vi "Send Notify Monitor.vi"(7 "Priority":T1 caption="Message Priority (Normal)", 8 "error in (no error)":errorcluster, 11 "Message Enqueuer in":refnum<class "Message Enqueuer.lvclass">) -> (0 "error out":errorcluster, 3 "Message Enqueuer out":refnum<class "Message Enqueuer.lvclass">)   [LabVIEW 2023, in "Monitored Actor.lvlib" / "Notify Monitor Msg.lvclass"]
doc: "Sends the <b>Monitored Actor.lvlib:Notify Monitor Msg.lvclass</b> message.\n\nThis message will call <b>Notify Monitor.vi</b> on the <b>Monitored Actor.lvlib:Monitored Actor.lvclass</b> actor.\n\n<b>Notify Monitor.vi Description</b>\nNotifies the actor monitor that a new actor has spawned\n\nCopyright: MGI 2016\nAuthor: Derek Trepanier"
uses:
  Notify Monitor Msg.lvclass
  builds/Engine/Actor Framework.lvlibp/1abvi3w/vi.lib/ActorFramework/Message Enqueuer/Message Enqueuer.lvclass
  builds/Engine/Actor Framework.lvlibp/1abvi3w/vi.lib/ActorFramework/Message Enqueuer/Message Priority.ctl
  C:/Users/Public/Documents/Development/builds/Engine/Actor Framework.lvlibp/1abvi3w/vi.lib/ActorFramework/Message/Message.lvclass
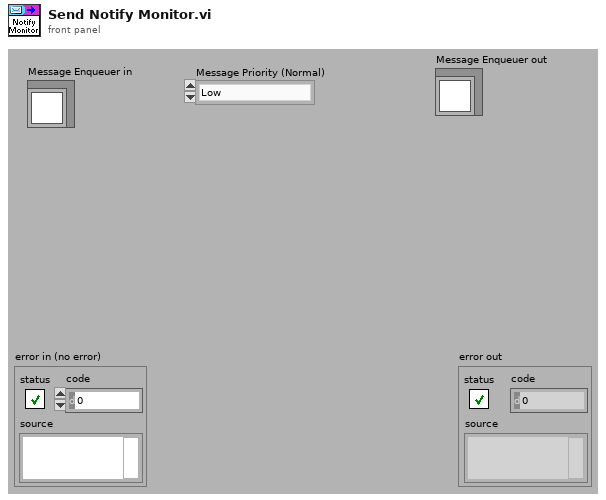
[diagram p1: front panel]
types:
  T1 = typedef "Actor Framework.lvlibp/Message Enqueuer.lvclass/Message Priority.ctl" = enum16{"Low", "Normal", "High"}
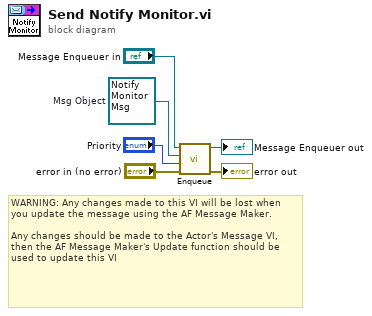
[diagram p0: block diagram]
diagram:
  w2 = refnum<class "Notify Monitor Msg.lvclass"> refnum  # Msg Object
  # "WARNING: Any changes made to this VI will be lost when you update the message using the AF Message Maker.\n\nAny changes should be made to the Actor's Message VI, then the AF Message Maker's Update function should be used to update this VI"
  n1 = call "Enqueue.vi"("error in (no error)"="error in (no error)", "Message Priority (Normal)"="Priority", "Message"=w2, "Message Enqueuer in"="Message Enqueuer in") -> ("error out"=→"error out":errorcluster, "Message Enqueuer out"=→"Message Enqueuer out":refnum<class "Message Enqueuer.lvclass">)  [unwired: 6 in]
